vi "create.vi"(8 "error in (no error)":errorcluster, 9 "size":i32, 10 "Image Type":T1 items=["Grayscale (U8)", "Grayscale (I16)", "Grayscale (SGL)", "Complex (CSG)", "RGB (U32)", "HSL (U32)", "RGB (U64)"], 11 "ImageCollection in":refnum<class "ImageCollection.lvclass">) -> (0 "error out":errorcluster, 3 "ImageCollection out":refnum<class "ImageCollection.lvclass">)   [LabVIEW 2010, in "ImageCollection.lvclass"]
uses:
  ImageCollection.lvclass
  Image/Image/Image.lvclass
  ImageCollection.lvclass/ImageCollection.ctl
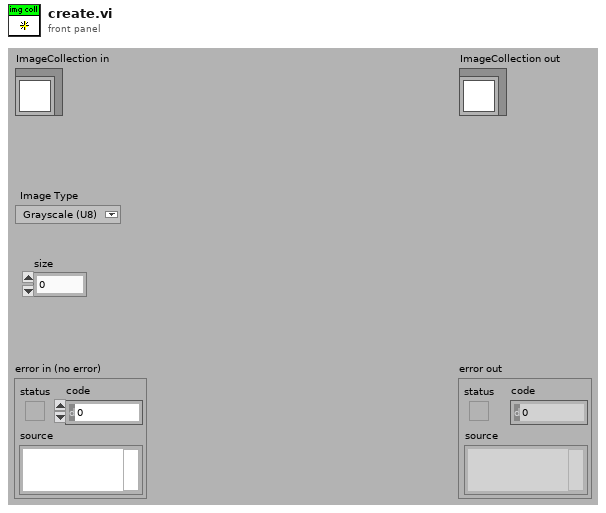
[diagram p1: front panel]
types:
  T1 = typedef "Image Type" = u32
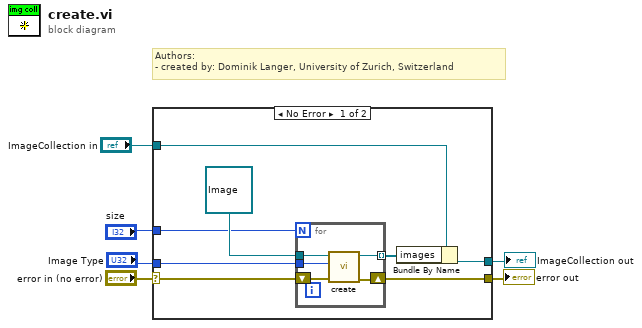
[diagram p0: block diagram]
diagram:
  # "Authors: \n- created by: Dominik Langer, University of Zurich, Switzerland"
  n1 = case shown="No Error" "error in (no error)" {
    selector: "error in (no error)" -> [w14 w21]
    tunnel: [w10 w21] -> w5
    tunnel: [w7 w20] -> w3
    tunnel: "ImageCollection in" -> [w8 w20]
    tunnel: "size" -> [w12 _]
    tunnel: "Image Type" -> [w11 _]
    frame No Error {
      n2 = for {
        N: w12 -> [_]
        tunnel: refnum<class "Image.lvclass"> refnum ("Image.lvclass") -> [w18]
        shift-right: [w17] -> w10
        shift-left: w14 -> [w19]
        tunnel: w11 -> [w16]
        tunnel: [w15] -> w9 mode=indexing
        n3 = call "create.vi"("error in (no error)"=w19, "Image Type"=w16, "Image in"=w18) -> ("error out"=w17:errorcluster, "Image out"=w15:refnum<class "Image.lvclass">)  [unwired: 1 in, 6 out]
      }
      n4 = Bundle By Name(cluster=w8, "images"=w9) -> (w7:refnum<class "ImageCollection.lvclass">)
    }
    frame Error {
    }
  }
  "error out" <- w5
  "ImageCollection out" <- w3
